vi "Digital (Pipelined Sample Clock) - Continuous Input.vi"() -> ()   [LabVIEW 2022 SP3]
doc: "This example demonstrates how to input a continuous digital waveform using pipelined sample clock mode. (An example of a device which is compatible with this timing type is a high speed source-synchronous ADC.)"
uses:
  <vilib>/Utility/error.llb/DialogType.ctl
  <vilib>/DAQmx/read.llb/DAQmx Read (Digital 1D Wfm NChan NSamp).vi
  <vilib>/DAQmx/create/channels.llb/DAQmx Create Channel (DI-Digital Input).vi
  <vilib>/DAQmx/configure/timing.llb/DAQmx Timing (Pipelined Sample Clock).vi
  <vilib>/DAQmx/miscellaneous.llb/DAQmx Fill In Error Info.vi
  <resource>/objmgr/daqmx.rc
panel:
  out "Digital Waveform Graph":digitalwaveform[](graph)
  in  "Samples per Buffer":u32=1000
  in  "Ready for Transfer \nDeassert Condition Threshold":i32=256
  in  "Ready for Transfer Output Terminal":tag="/Dev1/PFI0" caption="Ready for Transfer Output"
  in  "Ready for Transfer  Level":enum16{"Active High", "Active Low"}(ring)=enum."Active Low" caption="Ready for Transfer Level"
  in  "Handshaking?":bool
  in  "Pause Trigger Polarity (Pause When)":enum16{"High", "Low"}(ring)=enum."Low" caption="Pause Trigger Polarity"
  in  "Pause Trigger Source Terminal":tag="/Dev1/PFI1" caption="Pause Trigger Source"
  in  "Stop":bool
  in  "Sample Rate":dbl=1000.0
  in  "Line(s)":tag="Dev1/port0/line0:7"
  # "Channel Settings"
  # "Acquired Data"
  # "Timing Settings"
  # "Advanced Settings"
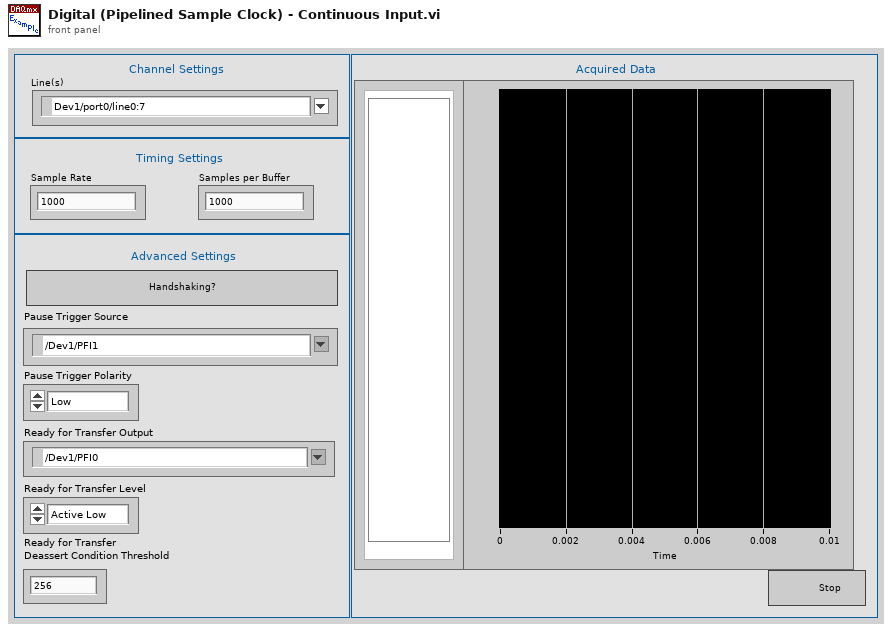
[diagram p1: front panel]
types:
  T1 = typedef "DialogType.ctl" = u16
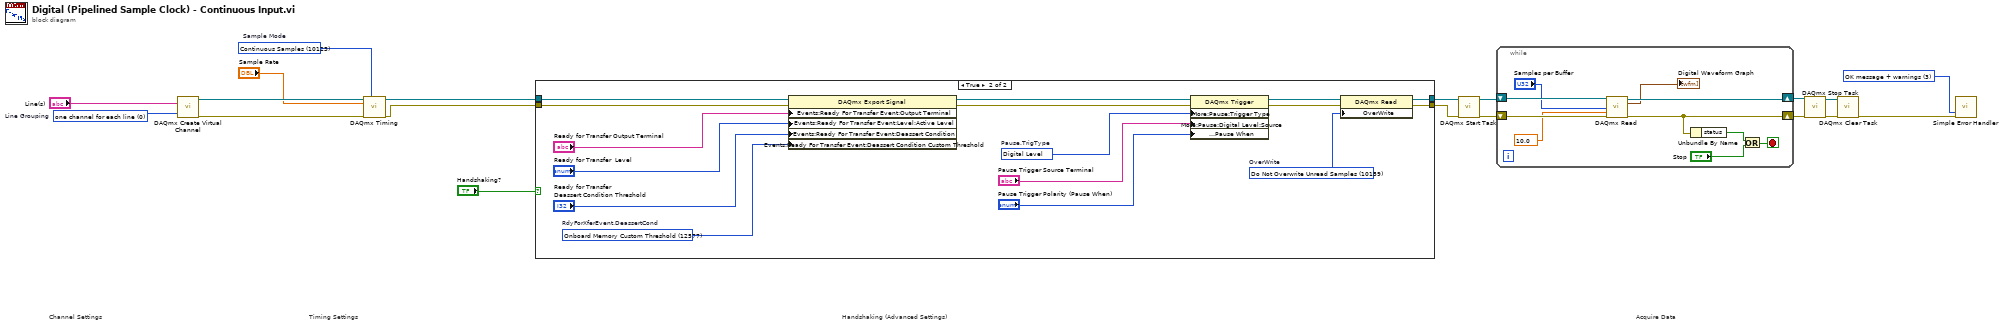
[diagram p0: block diagram]
diagram:
  w13 = T1 3 items=["no dialog", "OK message", "continue or stop message", "OK message + warnings", "continue/stop + warnings"] ("type of dialog (OK msg:1)")
  w17 = 10123 items=["Finite Samples"=10178, "Continuous Samples"=10123, "Hardware Timed Single Point"=12522]  # Sample Mode
  w19 = 0 items=["one channel for each line", "one channel for all lines"]  # Line Grouping
  # "Timing Settings"
  # "Acquire Data"
  # "Handshaking (Advanced Settings)"
  # "Channel Settings"
  n1 = call-poly <vilib>:"DAQmx Create Virtual Channel.vi"("lines"="Line(s)", "line grouping"=w19) -> ("task out"=w18:refnum<k21>, "error out"=w16:errorcluster)  [unwired: 12 in]
  n2 = call-poly <vilib>:"DAQmx Timing.vi"("task/channels in"=w18, "sample mode"=w17, "rate"="Sample Rate", "error in"=w16) -> ("task out"=w9:refnum<k21>, "error out"=w8:errorcluster)  [unwired: 10 in]
  n3 = case shown="True" "Handshaking?" {
    tunnel: [w20 w33] -> w6
    tunnel: [w21 w31] -> w7
    tunnel: w9 -> [w21 w28]
    tunnel: w8 -> [w20 w29]
    frame False {
    }
    frame True {
      w24 = 12577 items=["Onboard Memory More than Half Full"=10237, "Onboard Memory Full"=10236, "Onboard Memory Custom Threshold"=12577]  # RdyForXferEvent.DeassertCond
      w30 = 10159 items=["Overwrite Unread Samples"=10252, "Do Not Overwrite Unread Samples"=10159]  # OverWrite
      w37 = 10152 items=["Analog Level"=10101, "Analog Window"=10103, "Digital Level"=10152, "Digital Pattern"=10398, "None"=10230]  # Pause.TrigType
      n4 = property class="DAQmx Export Signal"(reference=w28, error in=w29, "Events:Ready For Transfer Event:Output Terminal"="Ready for Transfer Output Terminal", "Events:Ready For Transfer Event:Level:Active Level"="Ready for Transfer  Level", "Events:Ready For Transfer Event:Deassert Condition"="Ready for Transfer \nDeassert Condition Threshold", "Events:Ready For Transfer Event:Deassert Condition Custom Threshold"=w24) -> (reference out=w23:refnum<k21>, error out=w22:errorcluster)
      n5 = property class="DAQmx Trigger"(reference=w23, error in=w22, "More:Pause:Trigger Type"=w37, "More:Pause:Digital Level:Source"="Pause Trigger Source Terminal", "More:Pause:Digital Level:Pause When"="Pause Trigger Polarity (Pause When)") -> (reference out=w32:refnum<k21>, error out=w34:errorcluster)
      n6 = property class="DAQmx Read"(reference=w32, error in=w34, "OverWrite"=w30) -> (reference out=w31:refnum<k21>, error out=w33:errorcluster)
    }
  }
  n7 = call <vilib>:"DAQmx Start Task.vi"("task/channels in"=w7, "error in"=w6) -> ("task out"=w14:refnum<k21>, "error out"=w15:errorcluster)  [unwired: 12 in]
  n8 = while {
    shift-right: [w45] -> w2
    shift-left: w14 -> [w47]
    shift-right: [w44] -> w1
    shift-left: w15 -> [w46]
    stop <- w42 stop-if-true
    n9 = call-poly <vilib>:"DAQmx Read.vi"("task/channels in"=w47, "number of samples per channel"="Samples per Buffer", "timeout"=10.0, "error in"=w46) -> ("task out"=w45:refnum<k21>, "data"=→"Digital Waveform Graph":digitalwaveform[], "error out"=w44:errorcluster)  [unwired: 9 in]
    n10 = Unbundle By Name(w44) -> ("status"=w43:bool)
    n11 = Or(x=w43, y="Stop") -> (x .or. y?=w42:bool)
  }
  n12 = call <vilib>:"DAQmx Stop Task.vi"("task/channels in"=w2, "error in"=w1) -> ("task out"=w4:refnum<k21>, "error out"=w3:errorcluster)  [unwired: 12 in]
  n13 = call <vilib>:"DAQmx Clear Task.vi"("task in"=w4, "error in"=w3) -> ("error out"=w12:errorcluster)  [unwired: 13 in]
  n14 = call <vilib>:"Simple Error Handler.vi"("type of dialog (OK msg:1)"=w13, "error in (no error)"=w12) -> ()  [unwired: 3 in, 5 out]
